vi "DetectPulseIntervals.vi"(11 "Binary array probe":bool[](array[boolean])) -> (0 "Falling Index":i32[](array[numeric]), 1 "Rising Index":i32[](array[numeric]), 2 "Pulse lenghts out":i32[](array[numeric]), 3 "Interflank intervals out":i32[](array[numeric]), 4 "Pulse count out":u64)   [LabVIEW 2012]
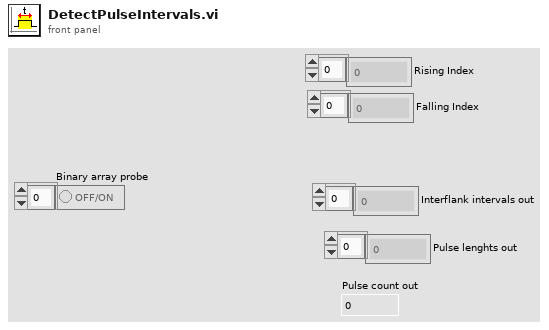
[diagram p1: front panel]
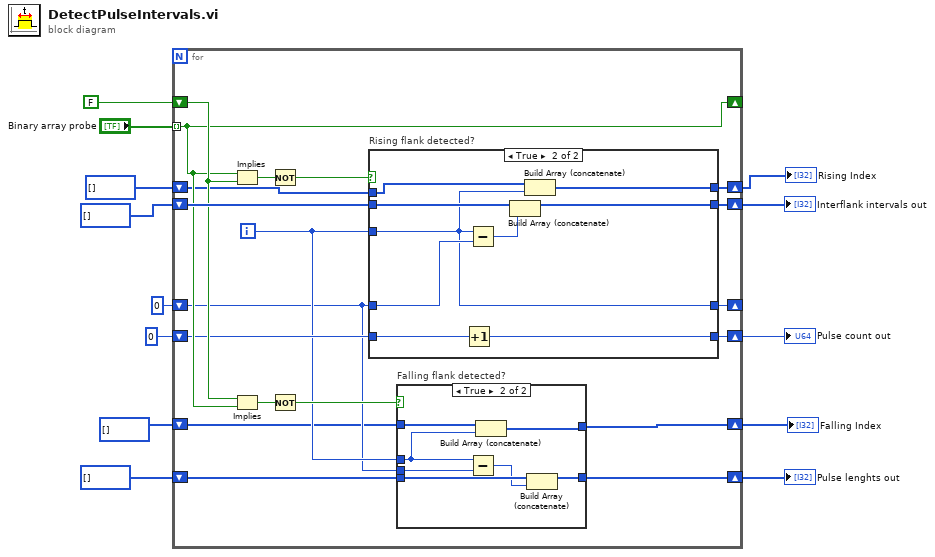
[diagram p0: block diagram]
diagram:
  n1 = for {
    tunnel: "Binary array probe" -> [w26] mode=indexing
    shift-right: [w26] -> _
    shift-left: FALSE ("Last reference value in") -> [w27]
    shift-right: [w30] -> _
    shift-left: 0 -> [w18]
    shift-right: [w29] -> w12
    shift-left: i32[] [] -> [w28]
    shift-right: [w22] -> w10
    shift-left: i32[] [] -> [w23]
    shift-right: [w20] -> w9
    shift-left: u64 0 ("Pulse count in") -> [w21]
    shift-right: [w14] -> w1
    shift-left: i32[] [] -> [w16]
    shift-right: [w15] -> w2
    shift-left: i32[] [] -> [w17]
    i -> [w19]
    n2 = Implies(1:w27, 2:w26) -> (0:w32:bool)
    n3 = Implies(1:w26, 2:w27) -> (0:w25:bool)
    n4 = Not(x=w32) -> (.not. x?=w31:bool)
    n5 = Not(x=w25) -> (.not. x?=w24:bool)
    n6 = case "Rising flank detected?" shown="True" w31 {
      tunnel: w19 -> [_ w46]
      tunnel: [w43 w46] -> w30
      tunnel: [w45 w54] -> w29
      tunnel: w28 -> [w45 w53]
      tunnel: w21 -> [w44 w52]
      tunnel: [w44 w51] -> w20
      tunnel: w18 -> [w43 w50]
      tunnel: w16 -> [w42 w48]
      tunnel: [w42 w47] -> w14
      frame False {
      }
      frame True {
        n7 = Increment(x=w52) -> (x+1=w51:u64)
        n8 = Subtract(x=w46, y=w50) -> (x-y=w49:i32)
        n9 = Build Array (concatenate)(w53, w49) -> (w54:i32[])
        n10 = Build Array (concatenate)(w48, w46) -> (w47:i32[])
      }
    }
    n11 = case "Falling flank detected?" shown="True" w24 {
      tunnel: w23 -> [w34 w41]
      tunnel: w19 -> [_ w37]
      tunnel: [w34 w39] -> w22
      tunnel: w18 -> [_ w38]
      tunnel: w17 -> [w33 w36]
      tunnel: [w33 w35] -> w15
      frame False {
      }
      frame True {
        n12 = Subtract(x=w37, y=w38) -> (x-y=w40:i32)
        n13 = Build Array (concatenate)(w36, w37) -> (w35:i32[])
        n14 = Build Array (concatenate)(w41, w40) -> (w39:i32[])
      }
    }
  }
  "Pulse count out" <- w9
  "Interflank intervals out" <- w12
  "Pulse lenghts out" <- w10
  "Falling Index" <- w2
  "Rising Index" <- w1
